vi "Do.vi"(8 "error in (no error)":errorcluster, 10 "Actor in":refnum<class "Actor.lvclass">, 11 "PV-Update Msg":refnum<class "PV-Update Msg.lvclass">) -> (0 "error out":errorcluster, 2 "Actor out":refnum<class "Actor.lvclass">)   [LabVIEW 2014, in "CS++DIM-Client.lvlib" / "PV-Update Msg.lvclass"]
doc: "(<B>Filename</B>: Actor Framework.lvlib:Message.lvclass:Do.vi)\n\nDefines what a message does when it is received by an actor. Generally, a message instructs an actor to invoke one of its methods.\n\nBy default, this method does nothing. A child class must override it to define behavior. Create a child class by using the Actor Framework Message Maker dialog box."
uses:
  PV-Update Msg.lvclass
  <vilib>/ActorFramework/Actor/Actor.lvclass
  CS++DIM-Client/CS++DIM-Client.lvclass
  CSPP_Core/Actors/CS++PVMonitor Messages/CS++PVUpdate Msg/CS++PVUpdate Msg.lvclass/CS++PVUpdate Msg.ctl
  CSPP_Core/Classes/CS++ProcessVariables/ProcessVariable/PV.lvclass
  CSPP_Core/Actors/CS++PVMonitor Messages/CS++PVUpdate Msg/CS++PVUpdate Msg.lvclass
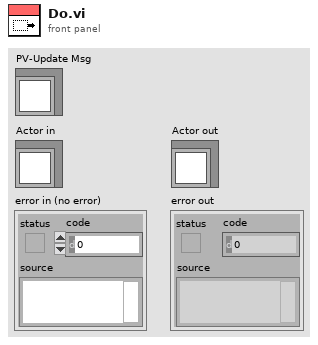
[diagram p1: front panel]
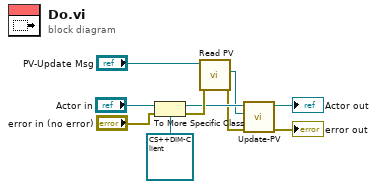
[diagram p0: block diagram]
diagram:
  n1 = To More Specific Class(target class=refnum<class "CS++DIM-Client.lvclass"> refnum ("CS++DIM-Client.lvlib:CS++DIM-Client.lvclass"), reference="Actor in", error in="error in (no error)") -> (specific class reference=w5:refnum<class "CS++DIM-Client.lvclass">, error out=w10:errorcluster)
  n2 = call "Read PV.vi"("error in (no error)"=w10, "CS++PVUpdate Msg in"="PV-Update Msg") -> ("error out"=w4:errorcluster, "PV"=w3:refnum<class "PV.lvclass">)  [unwired: 7 in, 1 out]
  n3 = call "Update-PV.vi"("error in (no error)"=w4, "PV"=w3, "CS++DIM-Client in"=w5) -> ("error out"=→"error out":errorcluster, "CS++DIM-Client out"=→"Actor out":refnum<class "CS++DIM-Client.lvclass">)  [unwired: 7 in]
